vi "불리언 연산.vi"() -> ()   [LabVIEW 2020]
panel:
  out "불리언을 숫자로 변환":dbl
  out "결과":bool
  in  "C":bool
  in  "B":bool
  in  "A":bool
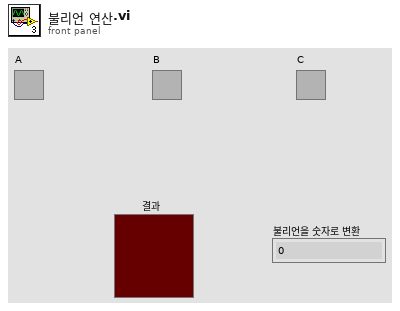
[diagram p1: front panel]
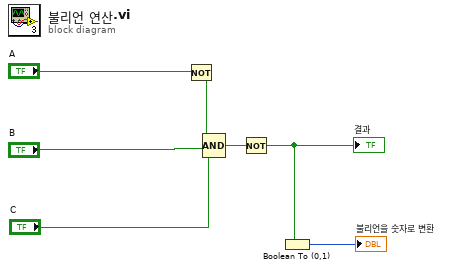
[diagram p0: block diagram]
diagram:
  n1 = Not(x="A") -> (.not. x?=w2:bool)
  n2 = Compound Arithmetic op=AND(w2, "B", "C") -> (w4:bool)
  n3 = Not(x=w4) -> (.not. x?=w1:bool)
  "결과" <- w1
  n4 = Boolean To (0,1)(Boolean=w1) -> (0, 1=→"불리언을 숫자로 변환":i16)
